vi "Enqueuer.vi"(6 "Priority Message? (F)":bool, 7 "Start Time":timestamp, 8 "error in (no error)":errorcluster, 9 "Message Data":variant, 10 "Message":string, 11 "Queue":refnum<queue>) -> (0 "error out":errorcluster)   [LabVIEW 2020, in "Scheduled Enqueue.lvclass"]
uses:
  Scheduled Enqueue.lvclass
  support/Message Queue/Message Cluster.ctl
  <vilib>/Platform/TimedLoop/XDataNode/timing_clust.ctl
  <vilib>/Platform/TimedLoop/XDataNode/nitl_modes.ctl
  <vilib>/Platform/TimedLoop/XDataNode/wakeup.ctl
  <vilib>/Platform/TimedLoop/TimeConversion.llb/rt-timestamp-to-milliseconds.vi
  support/Message Queue/Enqueue Message (Single).vi
  <vilib>/platform/TimedLoop/XDataNode/XDataNode.xnode
  Scheduled Enqueue.lvclass/Scheduled Enqueue.ctl
  <vilib>/Platform/TimedLoop/XDataNode/XDNodeRunTimeDep.lvlib
  support/Message Queue/Message Queue.lvlib
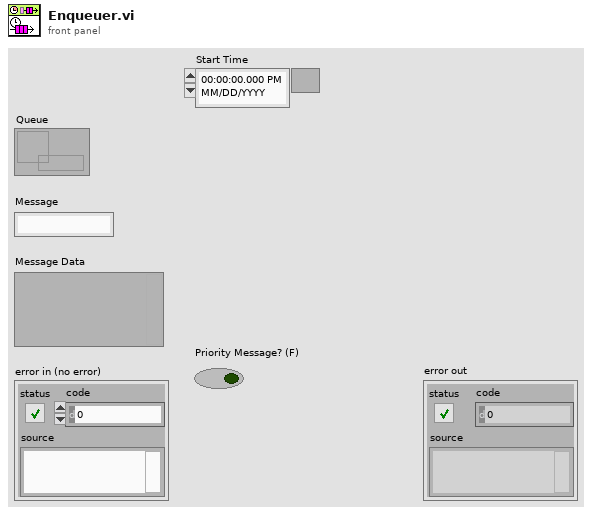
[diagram p1: front panel]
types:
  T1 = typedef "XDNodeRunTimeDep.lvlib/timing_clust.ctl" = cluster{"Expected End [f-1]":u64, "Actual End [f-1]":u64, "Finished Late? [f-1]":bool, "Expected End [i-1]":u64, "Actual End [i-1]":u64, "Finished Late? [i-1]":bool, "Expected Start [i]":u64, "Actual Start [i]":u64, "Expected Start [f]":u64, "Actual Start [f]":u64, "Source Name":string, "Structure Name":string, "Period":i64, "Deadline":i64, "Offset":i64, "Start":i64, "Priority":i32, "Timeout":i32, "Mode":T2, "Wakeup Reason":T3, "Error":errorcluster, "Source Type":string, "Secondary Source Type":string, "Global End Time":u64, "Global Start Time":u64, "Frame Duration":u64, "Iteration Duration":u64, "Assigned CPU":i32, "I/O Scan Engine Mode":u32}
  T2 = typedef "XDNodeRunTimeDep.lvlib/nitl_modes.ctl" = enum32{"No Change", "Process missed periods, maintain original phase", "Discard missed periods, maintain original phase", "Process missed periods, ignore original phase", "Discard missed periods, ignore original phase"}
  T3 = typedef "XDNodeRunTimeDep.lvlib/wakeup.ctl" = enum32{"Normal", "Aborted", "Asynchronous wakeup", "Timing source error", "Timed loop error", "Timeout"}
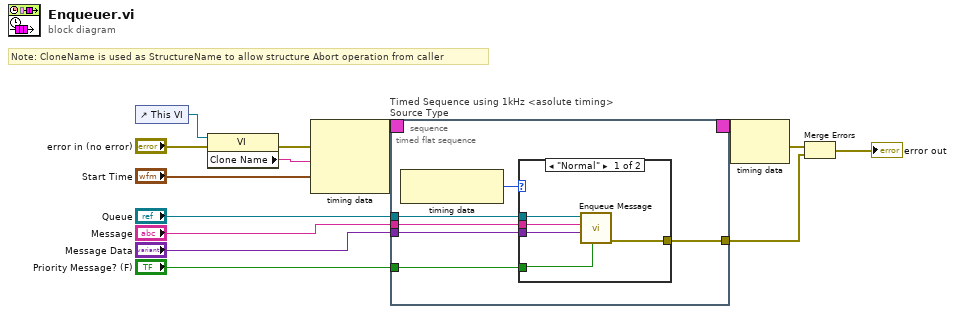
[diagram p0: block diagram]
diagram:
  # "Note: CloneName is used as StructureName to allow structure Abort operation from caller"
  n1 = control-ref of="This VI"() -> (w12:refnum<vi>)
  n2 = property class="VI"(reference=w12, error in="error in (no error)") -> (error out=w8:errorcluster, "Clone Name"=w7:string)  [unwired: 1 out]
  n3 = node-c288(w8, w7, "Start Time") -> (w14:T1)
  n4 = timed-sequence "Timed Sequence using 1kHz <asolute timing> Source Type" {
    timing: w14 -> [_]
    timing-out: [_] -> w13
    tunnel: "Queue" -> [w19]
    tunnel: "Message" -> [w18]
    tunnel: "Message Data" -> [w17]
    tunnel: [w16] -> w4
    tunnel: "Priority Message? (F)" -> [w15]
    n5 = timed-flat-sequence {
      tunnel: w19 -> [w25]
      tunnel: w18 -> [w23]
      tunnel: w17 -> [w22]
      tunnel: [w21] -> w16
      tunnel: w15 -> [w20]
      n6 = node-c288() -> (w24:T3)  [unwired: 1 in]
      n7 = case shown="\"Normal\"" w24 {
        tunnel: w25 -> [w30 _]
        tunnel: w23 -> [w29 _]
        tunnel: w22 -> [w28 _]
        tunnel: [w27 _] -> w21
        tunnel: w20 -> [w26 _]
        frame "Normal" {
          n8 = call-poly "Enqueue Message.vi"("Priority Message? (F)"=w26, "Message Data"=w28, "Message"=w29, "Message Queue"=w30) -> ("error out"=w27:errorcluster)  [unwired: 6 in, 1 out]
        }
        frame "Aborted", Default {
        }
      }
    }
  }
  n9 = node-c288(w13) -> (w5:errorcluster)
  n10 = Merge Errors(w5, w4) -> (→"error out":errorcluster)
